vi "pcc_3ch.vi"() -> ()   [LabVIEW 2020]
uses:
  C:/Program Files/Dotfast Consulting/Timetag Explorer 2.26/ttInterface.dll
  Program Files/Dotfast Consulting/Timetag Explorer 2.26/ttInterface.dll
panel:
  out "Waveform Chart":T1(graph)
  in  "stop":bool
  out "Acq Time":dbl
  in  "Iterations":i32
  out "Array":i32[](array[numeric])
  in  "Cycle Time":dbl=1.0 caption="Delay Time (s)"
  in  "Ctw(ns)":dbl
  in  "S2b":u8
  in  "S2p":u8
  in  "S1b":u8
  in  "S1p":u8
  in  "R":u8
  in  "Ch Array":u8[](array[numeric]) caption="Ch"
  in  "Ch Delay (ns)":dbl[](array[numeric])
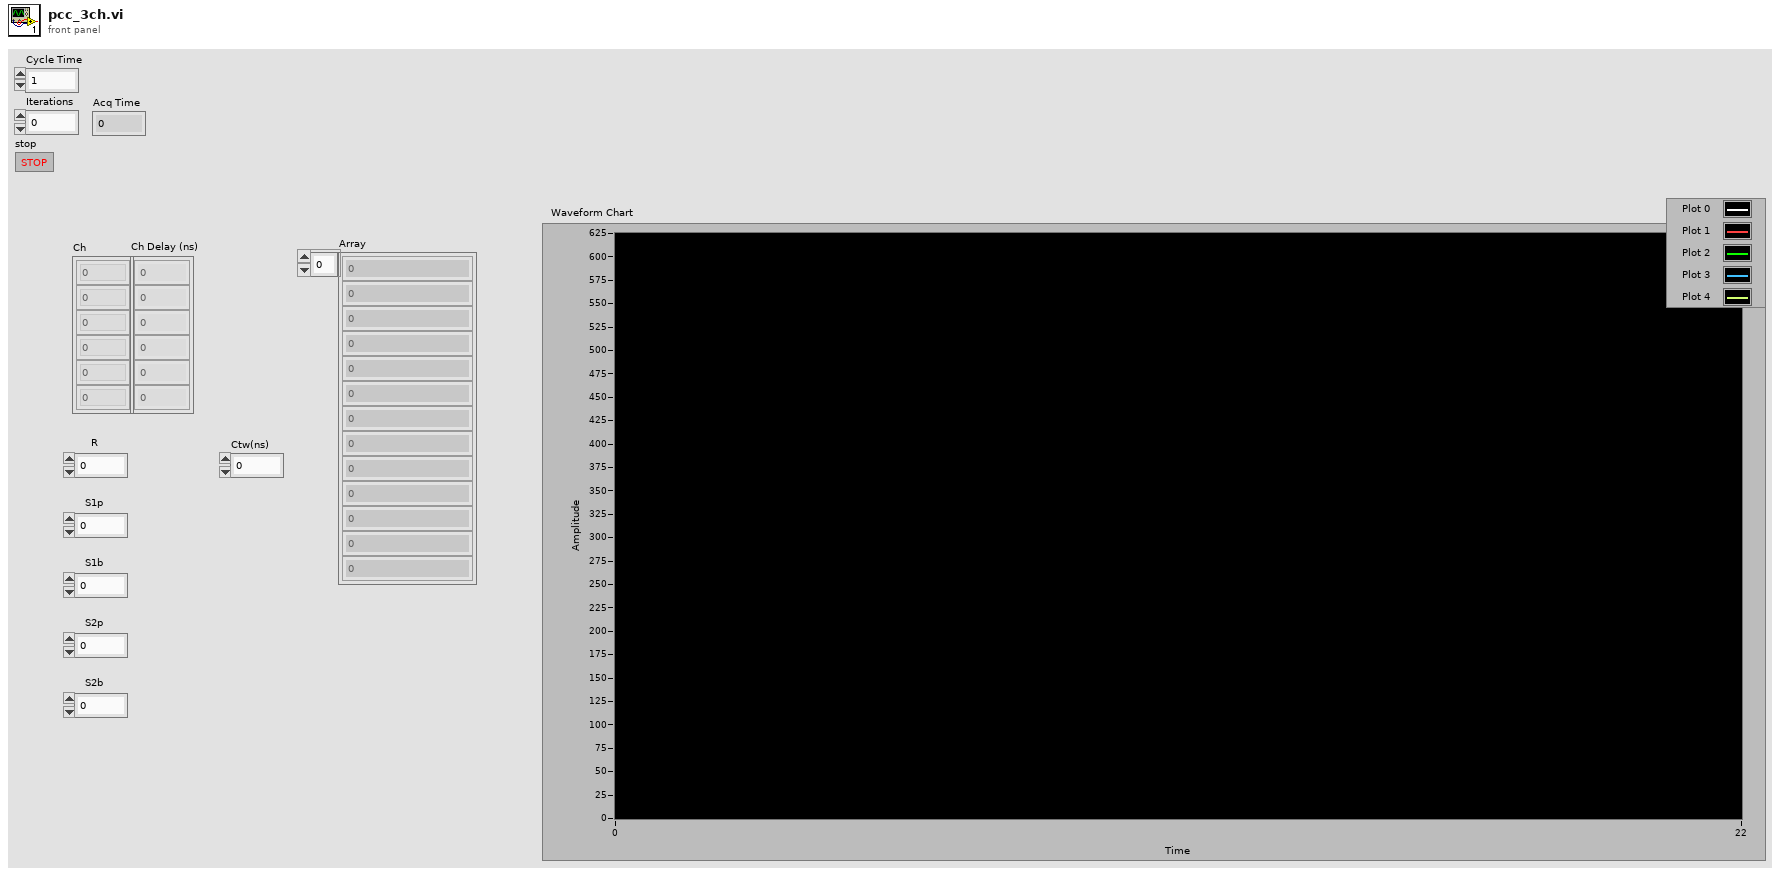
[diagram p1: front panel]
types:
  T1 = cluster{"[0]":i32, "[1]":i32, "[2]":i32, "[3]":i32, "[4]":i32, "[5]":i32, "[6]":i32, "[7]":i32, "[8]":i32}
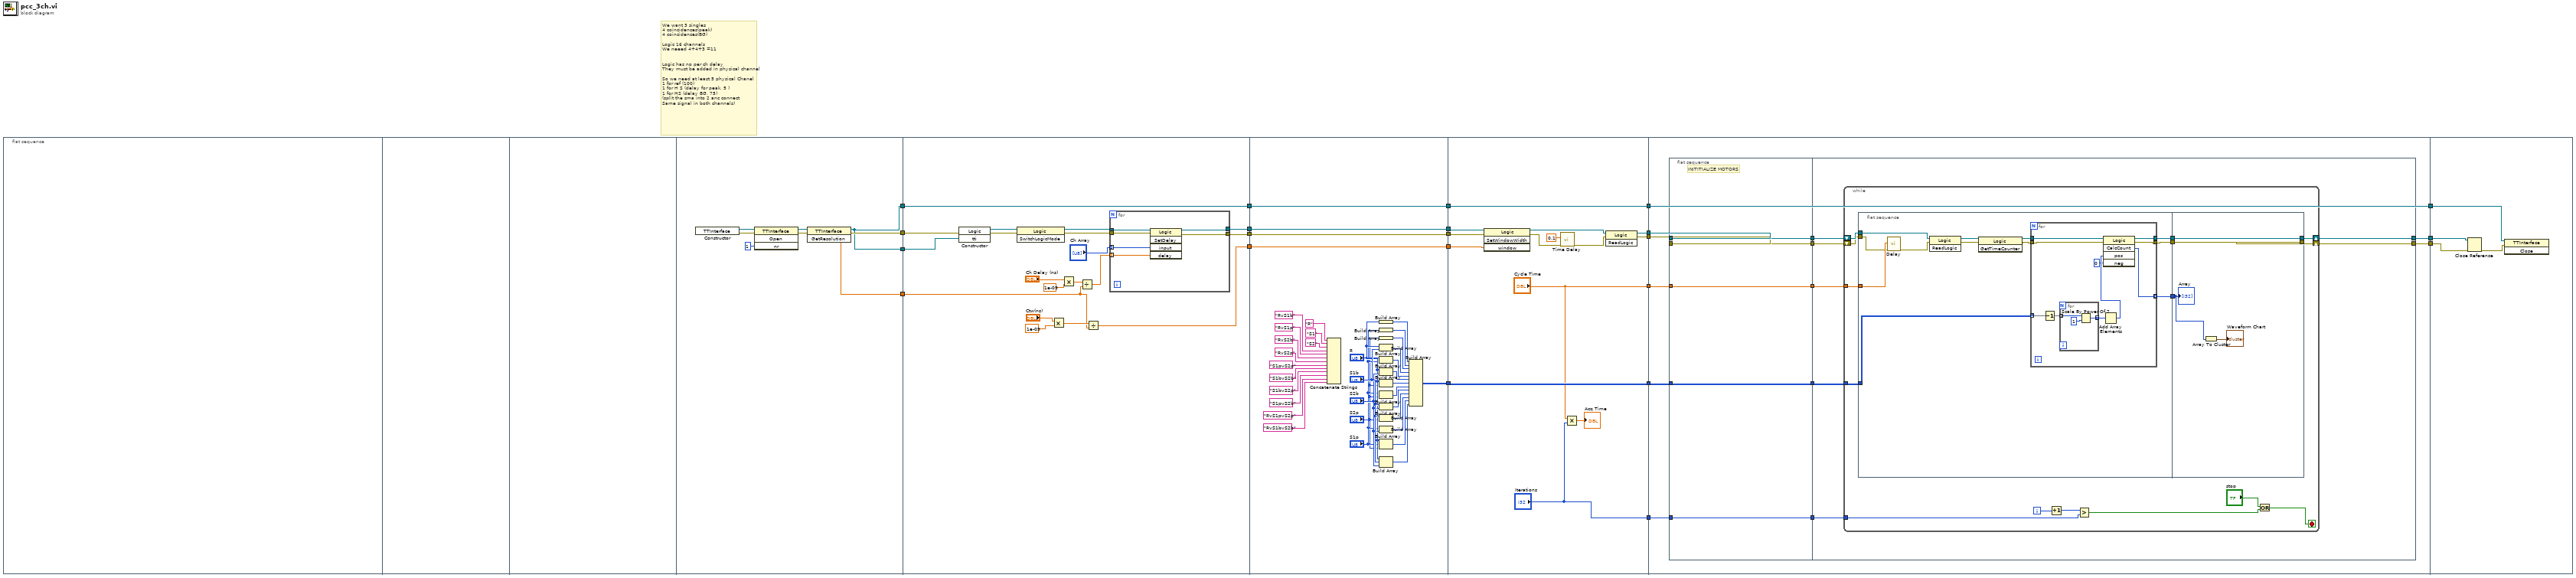
[diagram p0: block diagram]
diagram:
  # "We want 3 singles\n4 coincidences(peak)\n4 coincidences(BG)\n\nLogic 16 channels\nWe neeed 4+4+3 =11\n\n\nLogic has no per ch delay\nThey must be added in physical channel\n\nSo we need at least 5 physical Chanel\n1 for ref (100)\n1 for H S (delay for peak, 5 )\n1 for HS (delay BG, 75)\n(split the sma into 2 anc connect\nSame signal in both channels)"
  n1 = flat-sequence {
    tunnel: [w23] -> w22
    tunnel: [w25] -> w21
    tunnel: [w24] -> w20
    tunnel: [w23] -> w6
    tunnel: w22 -> [w49]
    tunnel: w21 -> [w48]
    tunnel: w20 -> [w33]
    tunnel: [w38] -> w19
    tunnel: [w37] -> w18
    tunnel: [w32] -> w13
    tunnel: w6 -> [w31]
    tunnel: [w31] -> w5
    tunnel: w19 -> [w60]
    tunnel: w18 -> [w59]
    tunnel: [w60] -> w17
    tunnel: [w59] -> w16
    tunnel: [w58] -> w15
    tunnel: [w57] -> w14
    tunnel: w13 -> [w57]
    tunnel: w5 -> [w56]
    tunnel: [w56] -> w4
    tunnel: w17 -> [w104]
    tunnel: w16 -> [w103]
    tunnel: w15 -> [w105]
    tunnel: w14 -> [w102]
    tunnel: [w105] -> w12
    tunnel: [w97] -> w11
    tunnel: [w96] -> w10
    tunnel: ["Cycle Time"] -> w9
    tunnel: w4 -> [w95]
    tunnel: [w95] -> w3
    tunnel: ["Iterations"] -> w1
    tunnel: w12 -> [w116]
    tunnel: w11 -> [w118]
    tunnel: w10 -> [w117]
    tunnel: w9 -> [w115]
    tunnel: [w114] -> w8
    tunnel: [w113] -> w7
    tunnel: w3 -> [w112]
    tunnel: [w112] -> w2
    tunnel: w1 -> [w111]
    tunnel: w8 -> [w178]
    tunnel: w7 -> [w177]
    tunnel: w2 -> [w176]
    frame #0 {
    }
    frame #1 {
    }
    frame #2 {
    }
    frame #3 {
      n2 = constructor class="TTInterface"() -> (reference out=w30:refnum<k24>, error out=w29:errorcluster)  [unwired: 3 in, 1 out]
      n3 = invoke class="TTInterface" method="Open"(reference=w30, error in=w29, "nr"=1) -> (reference out=w26:refnum<k24>, error out=w27:errorcluster)  [unwired: 1 in, 2 out]
      n4 = invoke class="TTInterface" method="GetResolution"(reference=w26, error in=w27) -> (reference out=w23:refnum<k24>, error out=w25:errorcluster, "GetResolution"=w24:dbl)  [unwired: 1 in]
    }
    frame #4 {
      n5 = constructor class="Logic"(error in=w48, "tti"=w49) -> (reference out=w47:refnum<k24>, error out=w46:errorcluster)  [unwired: 2 in, 2 out]
      n6 = invoke class="Logic" method="SwitchLogicMode"(reference=w47, error in=w46) -> (reference out=w45:refnum<k24>, error out=w44:errorcluster)  [unwired: 1 in, 1 out]
      n7 = Multiply(x="Ctw(ns)", y=1e-09) -> (x*y=w34:dbl)
      n8 = Multiply(x="Ch Delay (ns)", y=1e-09) -> (x*y=w41:dbl[])
      n9 = Divide(x=w41, y=w33) -> (x/y=w40:dbl[])
      n10 = Divide(x=w34, y=w33) -> (x/y=w32:dbl)
      n11 = for {
        tunnel: w45 -> [w55]
        tunnel: w44 -> [w54]
        tunnel: w40 -> [w53] mode=indexing
        tunnel: "Ch Array" -> [w52] mode=indexing
        tunnel: [w51] -> w38
        tunnel: [w50] -> w37
        n12 = invoke class="Logic" method="SetDelay"(reference=w55, error in=w54, "input"=w52, "delay"=w53) -> (reference out=w51:refnum<k24>, error out=w50:errorcluster)  [unwired: 1 in, 3 out]
      }
    }
    frame #5 {
      n13 = Concatenate Strings("R" ("string"), "S1" ("string"), "S2" ("string"), "RvS1b" ("string"), "RvS1p" ("string"), "RvS2b" ("string"), "RvS2p" ("string"), "S1pvS2p" ("string"), "S1bvS2b" ("string"), "S1bvS2p" ("string"), "S1pvS2b" ("string"), "RvS1pvS2p" ("string"), "RvS1bvS2b" ("string")) -> ()  [unwired: 1 out]
      n14 = Build Array("R") -> (w65:u8[])
      n15 = Build Array("S1p") -> (w63:u8[])
      n16 = Build Array("S2p") -> (w61:u8[])
      n17 = Build Array("R", "S1b") -> (w79:u8[])
      n18 = Build Array("R", "S1p") -> (w78:u8[])
      n19 = Build Array("R", "S2b") -> (w77:u8[])
      n20 = Build Array("R", "S2p") -> (w76:u8[])
      n21 = Build Array("S1p", "S2p") -> (w75:u8[])
      n22 = Build Array("S1b", "S2b") -> (w74:u8[])
      n23 = Build Array("S1b", "S2p") -> (w73:u8[])
      n24 = Build Array("S1p", "S2b") -> (w72:u8[])
      n25 = Build Array("R", "S1p", "S2p") -> (w71:u8[])
      n26 = Build Array("R", "S1b", "S2b") -> (w70:u8[])
      n27 = Build Array(w65, w63, w61, w79, w78, w77, w76, w75, w74, w73, w72, w71, w70) -> (w58:u8[][])
    }
    frame #6 {
      n28 = invoke class="Logic" method="SetWindowWidth"(reference=w104, error in=w103, "window"=w102) -> (reference out=w99:refnum<k24>, error out=w100:errorcluster)  [unwired: 1 in, 2 out]
      n29 = call "Time Delay"("error in (no error)"=w100, "Delay Time (s)"=0.1) -> ("error out"=w98:errorcluster)  [unwired: 9 in]
      n30 = Multiply(x="Cycle Time", y="Iterations") -> (x*y=→"Acq Time":dbl)
      n31 = invoke class="Logic" method="ReadLogic"(reference=w99, error in=w98) -> (reference out=w97:refnum<k24>, error out=w96:errorcluster)  [unwired: 1 in, 1 out]
    }
    frame #7 {
      n32 = flat-sequence {
        tunnel: w111 -> [w119]
        tunnel: w115 -> [w120]
        tunnel: w116 -> [w121]
        tunnel: w117 -> [w122]
        tunnel: w118 -> [w123]
        tunnel: [w123] -> w110
        tunnel: [w122] -> w109
        tunnel: [w121] -> w108
        tunnel: [w120] -> w107
        tunnel: [w119] -> w106
        tunnel: [w126] -> w114
        tunnel: [w125] -> w113
        tunnel: w110 -> [w130]
        tunnel: w109 -> [w129]
        tunnel: w108 -> [w128]
        tunnel: w107 -> [w127]
        tunnel: w106 -> [w124]
        frame #0 {
          # "INITITIALIZE MOTORS"
        }
        frame #1 {
          n33 = while {
            tunnel: w128 -> [w140]
            tunnel: w127 -> [w139]
            shift-right: [w138] -> w126
            shift-left: w130 -> [w142]
            shift-right: [w137] -> w125
            shift-left: w129 -> [w141]
            tunnel: w124 -> [w134]
            i -> [w136]
            stop <- w132 stop-if-true
            n34 = flat-sequence {
              tunnel: w142 -> [w155]
              tunnel: w141 -> [w156]
              tunnel: w140 -> [w151]
              tunnel: w139 -> [w157]
              tunnel: [w148] -> w145
              tunnel: [w147] -> w144
              tunnel: [w146] -> w143
              tunnel: [w173] -> w137
              tunnel: [w174] -> w138
              tunnel: w145 -> [w174]
              tunnel: w144 -> [w173]
              tunnel: w143 -> [w172]
              frame #0 {
                n35 = call "Delay"("error in (no error)"=w156, "Delay Time (s)"=w157) -> ("error out"=w154:errorcluster)  [unwired: 9 in]
                n36 = invoke class="Logic" method="ReadLogic"(reference=w155, error in=w154) -> (reference out=w153:refnum<k24>, error out=w152:errorcluster)  [unwired: 1 in, 1 out]
                n37 = invoke class="Logic" method="GetTimeCounter"(reference=w153, error in=w152) -> (reference out=w150:refnum<k24>, error out=w149:errorcluster)  [unwired: 1 in, 1 out]
                n38 = for {
                  tunnel: w151 -> [w167] mode=indexing
                  tunnel: w150 -> [w163]
                  tunnel: w149 -> [w162]
                  tunnel: [w161] -> w148
                  tunnel: [w160] -> w147
                  tunnel: [w159] -> w146 mode=indexing
                  n39 = Decrement(x=w167) -> (x-1=w166:u8[])
                  n40 = for {
                    tunnel: w166 -> [w169] mode=indexing
                    tunnel: [w168] -> w165 mode=indexing
                    n41 = Scale By Power Of 2(n=w169, x=1) -> (x*2^n=w168:i32)
                  }
                  n42 = Add Array Elements(numeric array=w165) -> (sum=w164:i32)
                  n43 = invoke class="Logic" method="CalcCount"(reference=w163, error in=w162, "pos"=w164, "neg"=0) -> (reference out=w161:refnum<k24>, error out=w160:errorcluster, "CalcCount"=w159:i32)  [unwired: 1 in, 2 out]
                }
              }
              frame #1 {
                n44 = Array To Cluster(array=w172) -> (cluster=→"Waveform Chart":T1)
                "Array" <- w172
              }
            }
            n45 = Increment(x=w136) -> (x+1=w135:i32)
            n46 = Greater?(x=w135, y=w134) -> (0:w131:bool)
            n47 = Or(x="stop", y=w131) -> (x .or. y?=w132:bool)
          }
        }
      }
    }
    frame #8 {
      n48 = Close Reference(reference=w178, error in (no error)=w177) -> (error out=w175:errorcluster)
      n49 = invoke class="TTInterface" method="Close"(reference=w176, error in=w175) -> ()  [unwired: 1 in, 3 out]
    }
  }
